vi "XLSFormatter.vi"(8 "error in (no error)":errorcluster, 11 "Array":string[][](array[string])) -> (0 "error out":errorcluster, 3 "Array 2":string[][](array[string]))   [LabVIEW 2018, in "Controller.lvlib"]
uses:
  Controller.lvlib
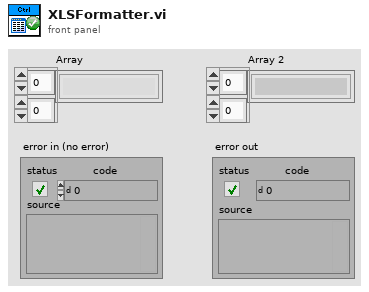
[diagram p1: front panel]
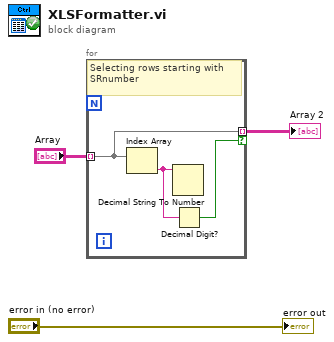
[diagram p0: block diagram]
diagram:
  n1 = for {
    tunnel: "Array" -> [w6] mode=indexing
    tunnel: [w6] -> w2 mode=indexing if=w4
    # "Selecting rows starting with SRnumber"
    n2 = Index Array(array=w6) -> (element=w5:string)  [unwired: 1 in]
    n3 = Decimal String To Number(string=w5) -> ()  [unwired: 2 in, 2 out]
    n4 = Decimal Digit?(1:w5) -> (0:w4:bool)
  }
  "Array 2" <- w2
  "error out" <- "error in (no error)"
